vi "MD5 format message-digest.vi"(8 "s4":u32 format="%.0x", 9 "s3":u32 format="%.0x", 10 "s2":u32 format="%.0x", 11 "s1":u32 format="%.0x") -> (3 "MD5 message-digest":string)   [LabVIEW 2011]
doc: "This VI performs certain bitwise operations on the state variables and converts them to hex strings such that they can be concatenated and displayed as the MD5 message-digest."
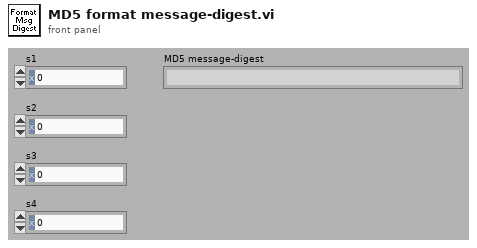
[diagram p1: front panel]
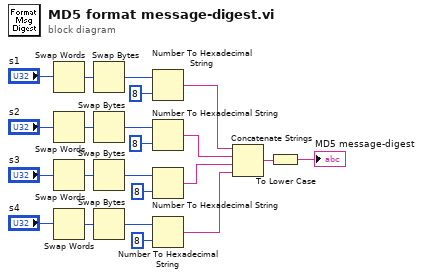
[diagram p0: block diagram]
diagram:
  n1 = Swap Words(1:"s1") -> (0:w20:u32)
  n2 = Swap Words(1:"s2") -> (0:w17:u32)
  n3 = Swap Words(1:"s3") -> (0:w13:u32)
  n4 = Swap Words(1:"s4") -> (0:w9:u32)
  n5 = Swap Bytes(anything=w20) -> (byte swapped=w19:u32)
  n6 = Swap Bytes(anything=w17) -> (byte swapped=w18:u32)
  n7 = Swap Bytes(anything=w13) -> (byte swapped=w12:u32)
  n8 = Swap Bytes(anything=w9) -> (byte swapped=w10:u32)
  n9 = Number To Hexadecimal String(1:i16 8 ("width (-)"), 2:w19) -> (0:w6:string)
  n10 = Number To Hexadecimal String(1:i16 8 ("width (-)"), 2:w18) -> (0:w5:string)
  n11 = Number To Hexadecimal String(1:i16 8 ("width (-)"), 2:w12) -> (0:w4:string)
  n12 = Number To Hexadecimal String(1:i16 8 ("width (-)"), 2:w10) -> (0:w3:string)
  n13 = Concatenate Strings(w6, w5, w4, w3) -> (w2:string)
  n14 = To Lower Case(string=w2) -> (all lower case string=→"MD5 message-digest":string)
